vi "identificationMAIN.vi"(7 "log?":bool) -> ()   [LabVIEW 2020]
uses:
  Qube/mode.ctl
  Qube/Qube.lvclass
panel:
  in  "refgen":cluster{"slope":dbl, "period (samples)":dbl}
  out "error":errorcluster
  in  "stop":bool
  out "u":dbl(graph)
  out "err":dbl(graph)
  out "dt":dbl(graph)
  out "y + r":cluster{"y":dbl, "y":dbl}(graph)
  # "1) Set the pathCtrl to the location of your\n     controller (the shared object .so)\n2) Set the pathDataCtrl to the location of \n     the controller data from MATLAB\n3) Press the white arrow near the top-left\n     corner. \n4) You can eventually log the data by\npressing \"Record\"."
  # "Change the slope and period value to see how your controller can track various ramps"
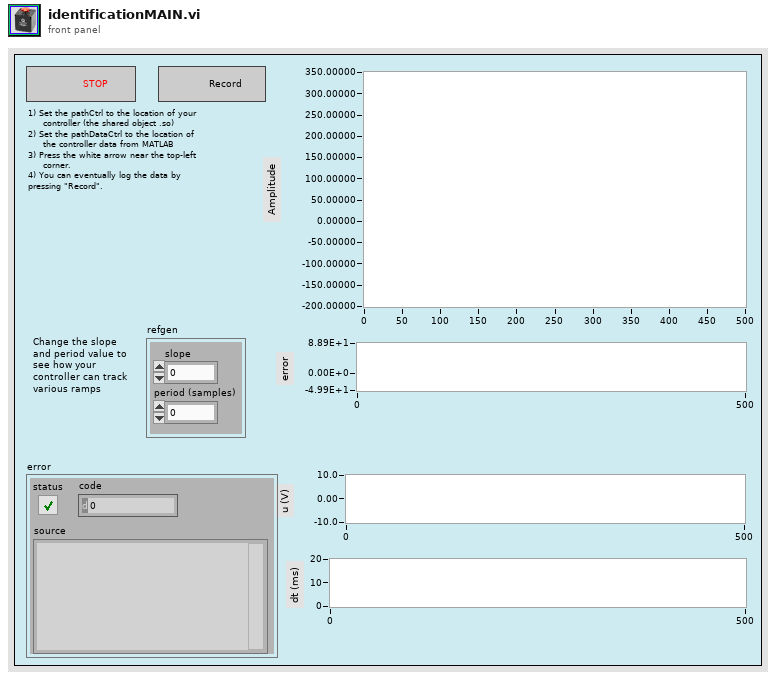
[diagram p1: front panel]
types:
  T1 = typedef "Qube.lvclass/mode.ctl" = enum16{"Control", "Identify"}
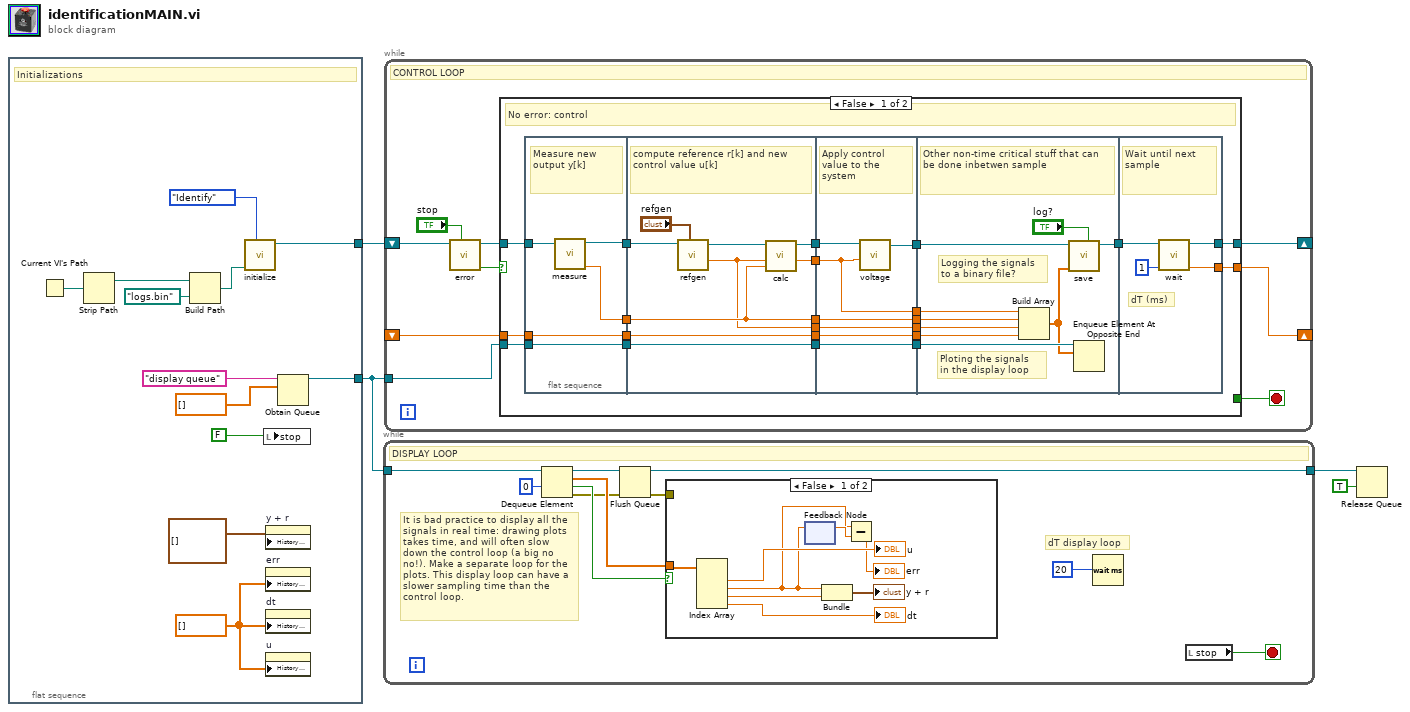
[diagram p0: block diagram]
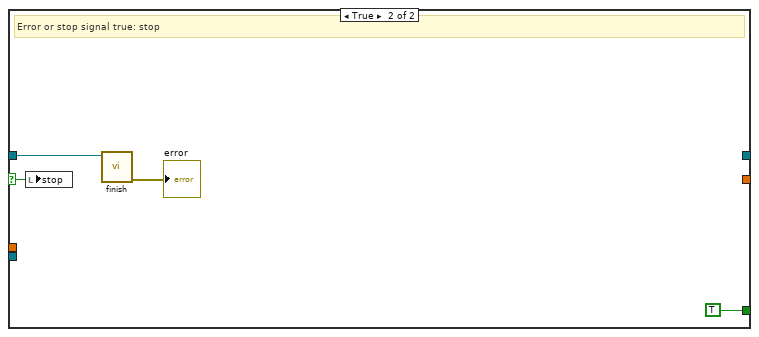
[diagram p3: hidden frame]
diagram:
  n1 = flat-sequence {
    tunnel: [w10] -> w4
    tunnel: [w16] -> w3
    frame #0 {
      w11 = dbl[] [] ("Waveform Chart")
      # "Initializations"
      n2 = Current VI's Path() -> (path=w9:path)
      n3 = Strip Path(path=w9) -> (stripped path=w8:path)  [unwired: 1 out]
      n4 = Build Path(base path=w8, name or relative path=path "logs.bin") -> (appended path=w6:path)
      n5 = call "initialize.vi"("mode"=mode."Identify", "log path"=w6) -> ("Qube"=w10:refnum<class "Qube.lvclass">)  [unwired: 9 in]
      n6 = local write "stop"(FALSE ("stop")) -> ()
      n7 = property on="y + r" class="WFChart (strict)"("History Data"=cluster{"y":dbl, "y":dbl}[] []) -> ()  [unwired: 2 in, 2 out]
      n8 = property on="err" class="WFChart (strict)"("History Data"=w11) -> ()  [unwired: 2 in, 2 out]
      n9 = property on="dt" class="WFChart (strict)"("History Data"=w11) -> ()  [unwired: 2 in, 2 out]
      n10 = property on="u" class="WFChart (strict)"("History Data"=w11) -> ()  [unwired: 2 in, 2 out]
      n11 = Obtain Queue(name (unnamed)="display queue", element data type=dbl[] [] ("y")) -> (queue out=w16:refnum<queue>)  [unwired: 3 in, 2 out]
    }
  }
  n12 = while {
    tunnel: w3 -> [w26]
    tunnel: [w18] -> w1
    stop <- w21 stop-if-true
    # "It is bad practice to display all the signals in real time: drawing plots takes time, and will often slow down the control loop (a big no no!). Make a separate loop for the plots. This display loop can have a slower sampling time than the control loop."
    # "dT display loop"
    # "DISPLAY LOOP"
    n13 = Dequeue Element(queue=w26, timeout in ms (-1)=0) -> (queue out=w22:refnum<queue>, element=w24:dbl[], timed out?=w25:bool, error out=w23:errorcluster)  [unwired: 1 in]
    n14 = Flush Queue(queue=w22, error in (no error)=w23) -> (queue out=w18:refnum<queue>, error out=w20:errorcluster)  [unwired: 1 out]
    n15 = case shown="False" w25 {
      tunnel: w24 -> [w34 _]
      tunnel: w20 -> [_ _]
      frame False {
        n16 = Index Array(array=w34) -> (element #1=→"u":dbl, element #2=w28:dbl, element #3=w31:dbl, element #4=→"dt":dbl)  [unwired: 4 in]
        n17 = feedback-in #1(w28) -> ()
        n18 = feedback #1() -> (w29:dbl)  [unwired: 1 in]
        n19 = Bundle("y"=w28, "y"=w31) -> (→"y + r":cluster{"y":dbl, "y":dbl})  [unwired: 1 in]
        n20 = Subtract(x=w28, y=w29) -> (x-y=→"err":dbl)
      }
      frame True {
      }
    }
    n21 = Wait (ms)(milliseconds to wait=u32 20 ("Ts")) -> ()  [unwired: 1 out]
    n22 = local read "stop"() -> (w21:bool)
  }
  n23 = while {
    shift-right: [w42] -> _
    shift-left: w4 -> [w36]
    tunnel: w3 -> [w41]
    shift-right: [w40] -> _
    shift-left: _ -> [w35]
    stop <- w43 stop-if-true
    # "CONTROL LOOP"
    n24 = call "error.vi"("stop"="stop", "Qube"=w36) -> ("abort?"=w38:bool, "Qube"=w39:refnum<class "Qube.lvclass">)  [unwired: 8 in]
    n25 = case shown="False" w38 {
      selector: w38 -> [_ w101]
      tunnel: w39 -> [w48 w102]
      tunnel: [_ TRUE] -> w43
      tunnel: [w62 _] -> w42
      tunnel: w41 -> [w59 _]
      tunnel: [w53 _] -> w40
      tunnel: w35 -> [w54 _]
      frame False {
        # "No error: control"
        n26 = flat-sequence {
          tunnel: w54 -> [w69]
          tunnel: w59 -> [w70]
          tunnel: [w66] -> w52
          tunnel: [w68] -> w51
          tunnel: [w70] -> w50
          tunnel: [w69] -> w49
          tunnel: w48 -> [w67]
          tunnel: [w76] -> w61
          tunnel: [w74] -> w60
          tunnel: [w79] -> w57
          tunnel: [w71] -> w55
          tunnel: w52 -> [w78]
          tunnel: w51 -> [w74]
          tunnel: w50 -> [w79]
          tunnel: w49 -> [w72]
          tunnel: [w73] -> w46
          tunnel: [w72] -> w45
          tunnel: [w86] -> w65
          tunnel: [w85] -> w63
          tunnel: w61 -> [w83]
          tunnel: w60 -> [w85]
          tunnel: [w84] -> w58
          tunnel: w57 -> [w84]
          tunnel: [w80] -> w56
          tunnel: w55 -> [w80]
          tunnel: [w82] -> w47
          tunnel: w46 -> [w82]
          tunnel: w45 -> [w81]
          tunnel: [w81] -> w44
          tunnel: w65 -> [w90]
          tunnel: [w95] -> w64
          tunnel: w63 -> [w94]
          tunnel: w58 -> [w92]
          tunnel: w56 -> [w89]
          tunnel: w47 -> [w88]
          tunnel: w44 -> [w87]
          tunnel: [w98] -> w62
          tunnel: w64 -> [w99]
          tunnel: [w96] -> w53
          frame #0 {
            # "Measure new output y[k]"
            n27 = call "measure.vi"("Qube"=w67) -> ("y"=w68:dbl, "Qube"=w66:refnum<class "Qube.lvclass">)  [unwired: 9 in]
          }
          frame #1 {
            # "compute reference r[k] and new control value u[k]"
            n28 = call "refgen.vi"("refgen"="refgen", "Qube"=w78) -> ("r"=w73:dbl, "Qube"=w77:refnum<class "Qube.lvclass">)  [unwired: 8 in]
            n29 = call "calc.vi"("y"=w74, "r"=w73, "Qube"=w77) -> ("u"=w71:dbl, "Qube"=w76:refnum<class "Qube.lvclass">)  [unwired: 7 in]
          }
          frame #2 {
            # "Apply control \nvalue to the system"
            n30 = call "voltage.vi"("u"=w80, "Qube"=w83) -> ("Qube"=w86:refnum<class "Qube.lvclass">)  [unwired: 9 in]
          }
          frame #3 {
            # "Ploting the signals\nin the display loop"
            # "Logging the signals to a binary file?"
            # "Other non-time critical stuff that can be done inbetwen sample"
            n31 = Build Array(w89, w94, w88, w87) -> (w91:dbl[])
            n32 = call "save.vi"("log?"="log?", "data"=w91, "Qube"=w90) -> ("Qube"=w95:refnum<class "Qube.lvclass">)  [unwired: 8 in]
            n33 = Enqueue Element At Opposite End(queue=w92, element=w91) -> ()  [unwired: 2 in, 3 out]
          }
          frame #4 {
            # "dT (ms)"
            # "Wait until next sample"
            n34 = call "wait.vi"("Ts (ms)"=u32 1, "Qube"=w99) -> ("dt"=w96:dbl, "Qube"=w98:refnum<class "Qube.lvclass">)  [unwired: 8 in]
          }
        }
      }
      frame True {
        # "Error or stop signal true: stop"
        n35 = local write "stop"(w101) -> ()
        n36 = call "finish.vi"("ActiveSuspension.lvclass"=w102) -> ("error out"=→"error":errorcluster)  [unwired: 10 in]
      }
    }
  }
  n37 = Release Queue(queue=w1, force destroy? (F)=TRUE) -> ()  [unwired: 1 in, 3 out]
